vi "dimensions.vi"() -> ()   [LabVIEW 2015, in "Get Object Parameters.xnode"]
uses:
  Get Object Parameters.xnode
panel:
  in  "header.h":i16=19
  in  "footer.h":i16=8
  in  "element.h":i16=19
  in  "resize.v":i32=19
  in  "min.h":i32=36
  in  "min.w":i32=32
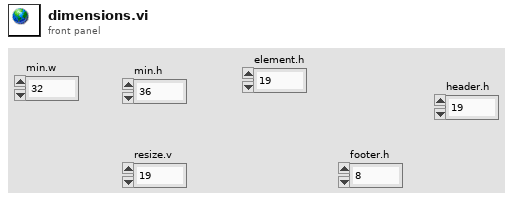
[diagram p1: front panel]
diagram:
